vi "Does_file_exist_(simple).vi"(1 "Pathname":path) -> (0 "exists?":bool)   [LabVIEW 2020]
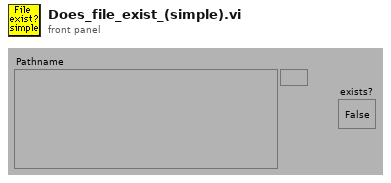
[diagram p1: front panel]
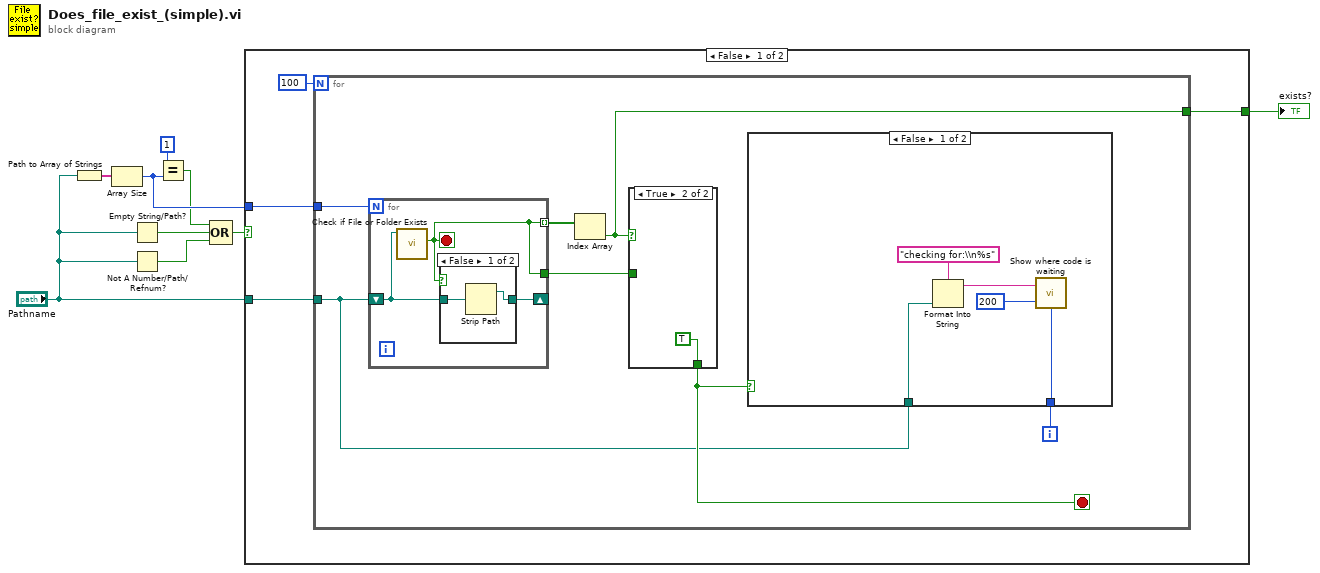
[diagram p0: block diagram]
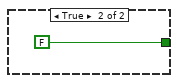
[diagram p5: hidden frame]
diagram:
  n1 = Path to Array of Strings(0:"Pathname") -> (2:w6:string[])  [unwired: 1 out]
  n2 = Array Size(array=w6) -> (size(s)=w4:i32)
  n3 = Empty String/Path?(string/path="Pathname") -> (empty?=w2:bool)
  n4 = Not A Number/Path/Refnum?(number/path/refnum="Pathname") -> (NaN/Path/Refnum?=w1:bool)
  n5 = Equal?(x=1, y=w4) -> (x = y?=w3:bool)
  n6 = Compound Arithmetic op=OR(w3, w2, w1) -> (w8:bool)
  n7 = case shown="False" w8 {
    tunnel: "Pathname" -> [w11 _]
    tunnel: [w12 FALSE ("file or folder exists?")] -> w9
    tunnel: w4 -> [w10 _]
    frame False {
      n8 = for {
        N: 100 -> [_]
        tunnel: w11 -> [w15]
        tunnel: [w17] -> w12
        tunnel: w10 -> [w16]
        i -> [w14]
        stop <- w18 stop-if-true
        n9 = for {
          N: w16 -> [_]
          tunnel: [w28] -> w20 mode=indexing
          shift-right: [w29] -> _
          shift-left: w15 -> [w30]
          tunnel: [w28] -> w19
          stop <- w28 stop-if-true
          n10 = call <vilib>:"Check if File or Folder Exists.vi"("path"=w30) -> ("file or folder exists?"=w28:bool)  [unwired: 1 in, 9 out]
          n11 = case shown="False" w28 {
            tunnel: w30 -> [w32 w33]
            tunnel: [w31 w33] -> w29
            frame False {
              n12 = Strip Path(path=w32) -> (stripped path=w31:path)  [unwired: 1 out]
            }
            frame True {
            }
          }
        }
        n13 = Index Array(array=w20) -> (element=w17:bool)  [unwired: 1 in]
        n14 = case shown="True" w17 {
          tunnel: w19 -> [w26 _]
          tunnel: [w26 TRUE] -> w18
          frame False {
          }
          frame True {
          }
        }
        n15 = case shown="False" w18 {
          tunnel: w15 -> [w24 _]
          tunnel: w14 -> [w21 _]
          frame False {
            n16 = Format Into String(format string="checking for:\\n%s", w24) -> (resulting string=w23:string)  [unwired: 2 in, 1 out]
            n17 = call "Show where code is waiting.vi"("Loop index"=w21, "Wait (ms)"=u32 200 ("milliseconds to wait"), "Message"=w23) -> ()  [unwired: 1 in]
          }
          frame True {
          }
        }
      }
    }
    frame True {
    }
  }
  "exists?" <- w9
